vi "FPGA_1WIRE_Write Byte.vi"(8 "error in":errorcluster, 10 "Tx data":u8) -> (0 "error out":errorcluster, 2 "Written":bool[](array[boolean]))   [LabVIEW 2020]
doc: "This VI is created by Vincent Claes for FPDA-1 more information on http://pwo.fpga.be\n\nvincent.claes@xios.be\nclaesvincent@gmail.com\n\nhttp://www.linkedin.com/in/vincentclaes"
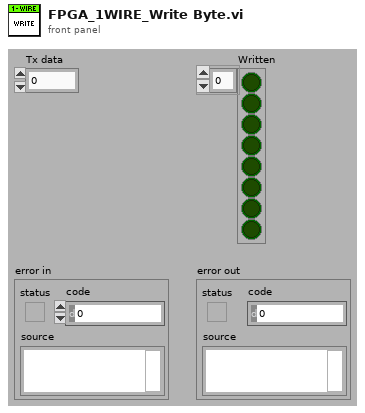
[diagram p1: front panel]
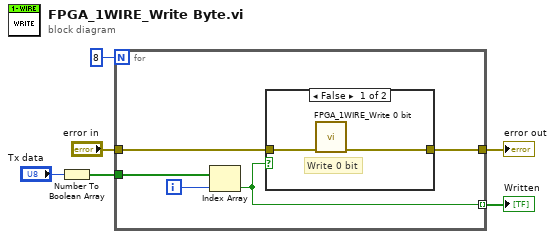
[diagram p0: block diagram]
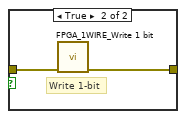
[diagram p2: hidden frame]
diagram:
  n1 = Number To Boolean Array(number="Tx data") -> (Boolean array=w6:bool[])
  n2 = for {
    N: 8 -> [_]
    tunnel: w6 -> [w11]
    tunnel: [w10] -> w3
    tunnel: "error in" -> [w9]
    tunnel: [w7] -> w1 mode=indexing
    i -> [w8]
    n3 = Index Array(array=w11, index=w8) -> (element=w7:bool)
    n4 = case shown="False" w7 {
      tunnel: [w12 w14] -> w10
      tunnel: w9 -> [w13 w15]
      frame False {
        # "Write 0 bit"
        n5 = call "FPGA_1WIRE_Write 0 bit.vi"("error in"=w13) -> ("error out"=w12:errorcluster)  [unwired: 10 in]
      }
      frame True {
        # "Write 1-bit"
        n6 = call "FPGA_1WIRE_Write 1 bit.vi"("error in"=w15) -> ("error out"=w14:errorcluster)  [unwired: 10 in]
      }
    }
  }
  "error out" <- w3
  "Written" <- w1
